vi "JJMCclase3.vi"() -> ()   [LabVIEW 2011]
panel:
  out "Alarma":string
  out "Observacion":string
  out "Alarma":bool
  out "Velocidad":i32(knob) scale=1.0..180.0
  out "Temperatura":dbl(slide) scale=0.0..100.0
  # "Generar la temperatura entre 1-100 y la velocidad entre 1-180 cuando la \nvelocidad sera mayor a 100 debemos escribir velocidad ALTA y cuando la temperatura\nsea mayor a 80 y la velocidad mayor a 120 se debe encender la alarma"
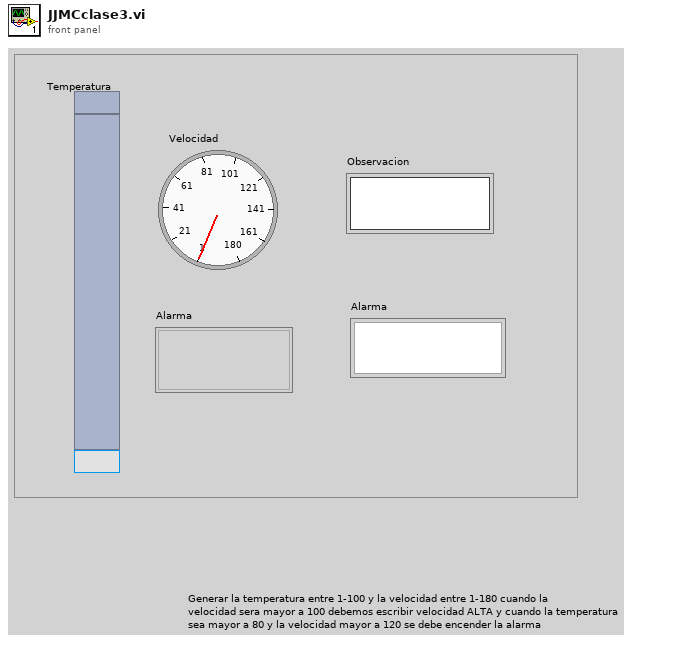
[diagram p1: front panel]
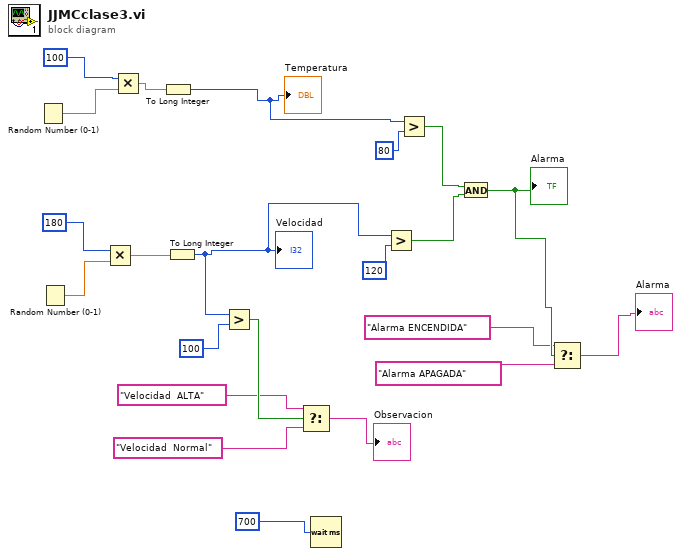
[diagram p0: block diagram]
diagram:
  n1 = Random Number (0-1)() -> (number: 0 to 1=w21:dbl)
  n2 = Random Number (0-1)() -> (number: 0 to 1=w7:dbl)
  n3 = Multiply(x=180, y=w7) -> (x*y=w19:dbl)
  n4 = Multiply(x=100, y=w21) -> (x*y=w20:dbl)
  n5 = To Long Integer(number=w20) -> (32bit integer=w14:i32)
  "Temperatura" <- w14
  n6 = To Long Integer(number=w19) -> (32bit integer=w10:i32)
  "Velocidad" <- w10
  n7 = Greater?(x=w10, y=100) -> (0:w17:bool)
  n8 = Select(t="Velocidad  ALTA", s=w17, f="Velocidad  Normal") -> (s? t:f=→"Observacion":string)
  n9 = Wait (ms)(milliseconds to wait=700) -> ()  [unwired: 1 out]
  n10 = Greater?(x=w10, y=120) -> (0:w9:bool)
  n11 = Greater?(x=w14, y=80) -> (0:w12:bool)
  n12 = And(x=w12, y=w9) -> (x .and. y?=w5:bool)
  "Alarma" <- w5
  n13 = Select(t="Alarma ENCENDIDA", s=w5, f="Alarma APAGADA") -> (s? t:f=→"Alarma":string)
